vi "SetClockSource.vi"(2 "error in (no error)":errorcluster, 3 "Clock Source":u16(ring) items=["Internal", "External"], 4 "VISA resource name":refnum<visa-resource-name>) -> (0 "error out":errorcluster, 1 "VISA resource name out":refnum<visa-resource-name>)   [LabVIEW 2020, in "Active Technologies AWG3000.lvlib"]
uses:
  Active Technologies AWG3000.lvlib
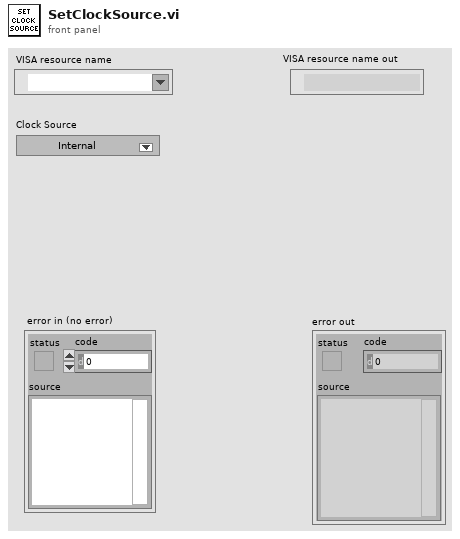
[diagram p1: front panel]
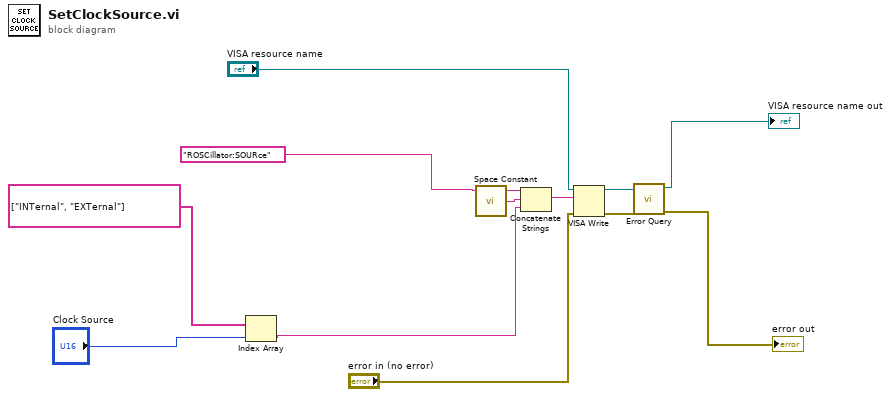
[diagram p0: block diagram]
diagram:
  n1 = Index Array(array=string[] ["INTernal", "EXTernal"], index="Clock Source") -> (element=w1:string)
  n2 = call <vilib>:"Space Constant.vi"() -> ("String"=w6:string)
  n3 = Concatenate Strings("ROSCillator:SOURce" ("write buffer"), w6, w1) -> (w5:string)
  n4 = VISA Write(VISA resource name="VISA resource name", write buffer=w5, error in (no error)="error in (no error)") -> (VISA resource name out=w10:refnum<visa-resource-name>, error out=w9:errorcluster)  [unwired: 1 out]
  n5 = call "Error Query.vi"("error in (no error)"=w9, "VISA resource name"=w10) -> ("error out"=→"error out":errorcluster, "VISA resource name out"=→"VISA resource name out":refnum<visa-resource-name>)  [unwired: 6 in, 2 out]
